vi "Define Folder Exclusion List.vi"(8 "error in (no error)":errorcluster, 11 "Test Executive Explorer in":refnum<class "Test Executive Explorer.lvclass">) -> (0 "error out":errorcluster, 3 "Test Executive Explorer out":refnum<class "Test Executive Explorer.lvclass">)   [LabVIEW 2017, in "Test Executive Explorer.lvclass"]
uses:
  Test Executive Explorer.lvclass
  <vilib>/gpm_packages/@cs/file-explorer-extension/Source/File Explorer/File Explorer/File Explorer.lvclass
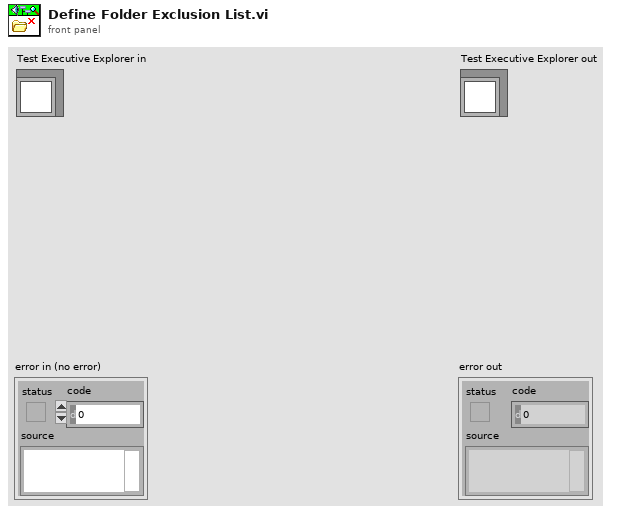
[diagram p1: front panel]
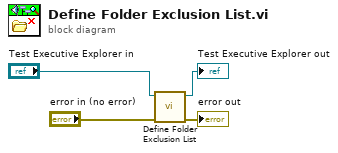
[diagram p0: block diagram]
diagram:
  n1 = call-parent "Define Folder Exclusion List.vi"("error in (no error)"="error in (no error)", "File Explorer in"="Test Executive Explorer in") -> ("error out"=→"error out":errorcluster, "File Explorer out"=→"Test Executive Explorer out":refnum<class "Test Executive Explorer.lvclass">)  [unwired: 8 in]
